vi "XY Graph Filter Plot Values.vi"(6 "Items to filter (Nan,+/-Inf)":dbl[](array[numeric])=[nan, inf, -inf], 10 "Y Array in":dbl[](array[numeric]), 11 "X Array in":dbl[](array[numeric])) -> (0 "Deleted Element Indices":i32[](array[numeric]), 2 "Y Array out":dbl[](array[numeric]), 3 "X Array out":dbl[](array[numeric]))   [LabVIEW 2021, in "XY Graph Add-Ons.lvlib"]
doc: "Removes points in a plot whose <b>Y</b> values are within the <b>Items to filter</b> array."
uses:
  XY Graph Add-Ons.lvlib
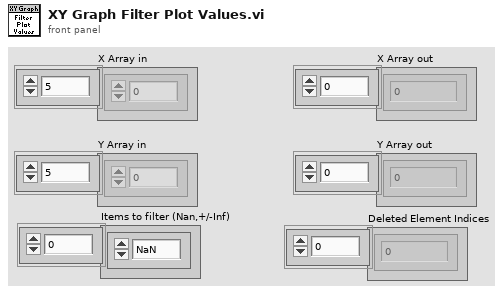
[diagram p1: front panel]
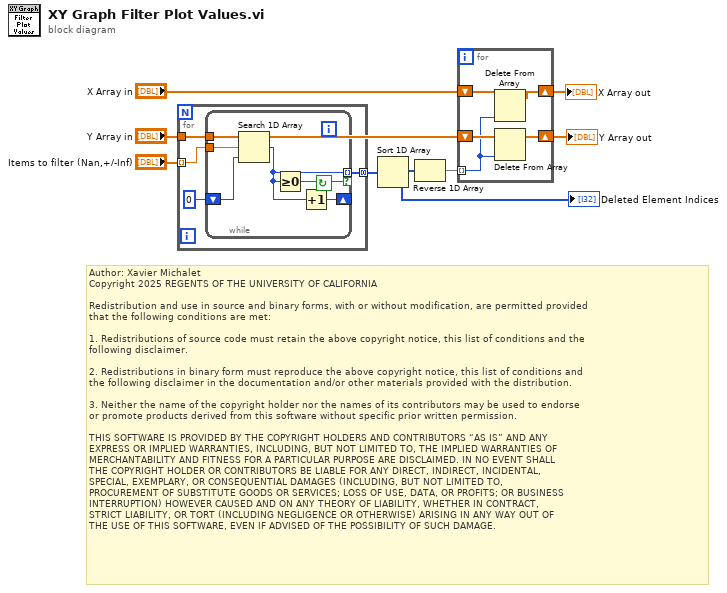
[diagram p0: block diagram]
diagram:
  # "Author: Xavier Michalet\nCopyright 2025 REGENTS OF THE UNIVERSITY OF CALIFORNIA\n\nRedistribution and use in source and binary forms, with or without modification, are permitted provided\nthat the following conditions are met:\n\n1. Redistributions of source code must retain the above copyright notice, this list of conditions and the\nfollowing disclaimer.\n\n2. Redistributions in binary form must reproduce the above copyright notice, this list of conditions and\nthe following disclaimer in the documentation and/or other materials provided with the distribution.\n\n3. Neither the name of the copyright holder nor the names of its contributors may be used to endorse \nor promote products derived from this software without specific prior written permission.\n\nTHIS SOFTWARE IS PROVIDED BY THE COPYRIGHT HOLDERS AND CONTRIBUTORS “AS IS” AND ANY \nEXPRESS OR IMPLIED WARRANTIES, INCLUDING, BUT NOT LIMITED TO, THE IMPLIED WARRANTIES OF\nMERCHANTABILITY AND FITNESS FOR A PARTICULAR PURPOSE ARE DISCLAIMED. IN NO EVENT SHALL\nTHE COPYRIGHT HOLDER OR CONTRIBUTORS BE LIABLE FOR ANY DIRECT, INDIRECT, INCIDENTAL, \nSPECIAL, EXEMPLARY, OR CONSEQUENTIAL DAMAGES (INCLUDING, BUT NOT LIMITED TO, \nPROCUREMENT OF SUBSTITUTE GOODS OR SERVICES; LOSS OF USE, DATA, OR PROFITS; OR BUSINESS\nINTERRUPTION) HOWEVER CAUSED AND ON ANY THEORY OF LIABILITY, WHETHER IN CONTRACT, \nSTRICT LIABILITY, OR TORT (INCLUDING NEGLIGENCE OR OTHERWISE) ARISING IN ANY WAY OUT OF\nTHE USE OF THIS SOFTWARE, EVEN IF ADVISED OF THE POSSIBILITY OF SUCH DAMAGE."
  n1 = for {
    tunnel: "Items to filter (Nan,+/-Inf)" -> [w11] mode=indexing
    tunnel: "Y Array in" -> [w12]
    tunnel: [w9] -> w7 mode=concatenating
    n2 = while {
      shift-right: [w15] -> _
      shift-left: 0 ("Start Index (0)") -> [w18]
      tunnel: w12 -> [w17]
      tunnel: w11 -> [w16]
      tunnel: [w14] -> w9 mode=indexing if=w13
      stop <- w13 continue-if-true
      n3 = Search 1D Array(1D array=w17, element=w16, start index (0)=w18) -> (index of element=w14:i32)
      n4 = Greater Or Equal To 0?(x=w14) -> (x >= 0?=w13:bool)
      n5 = Increment(x=w14) -> (x+1=w15:i32)
    }
  }
  n6 = Sort 1D Array(array=w7) -> (sorted array=w1:i32[])
  "Deleted Element Indices" <- w1
  n7 = Reverse 1D Array(array=w1) -> (reversed array=w6:i32[])
  n8 = for {
    tunnel: w6 -> [w20] mode=indexing
    shift-right: [w22] -> w3
    shift-left: "X Array in" -> [w23]
    shift-right: [w19] -> w2
    shift-left: "Y Array in" -> [w21]
    n9 = Delete From Array(array=w23, index=w20) -> (array with subset deleted=w22:dbl[])  [unwired: 1 in, 1 out]
    n10 = Delete From Array(array=w21, index=w20) -> (array with subset deleted=w19:dbl[])  [unwired: 1 in, 1 out]
  }
  "Y Array out" <- w2
  "X Array out" <- w3
